vi "LaunchMazeUI.vi"   [LabVIEW 2020]
panel:
  # "Loading Maze UI..."
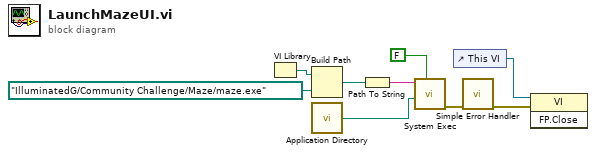
[diagram p0: block diagram]
diagram:
  n1 = VI Library() -> (path=w9:path)
  n2 = Build Path(base path=w9, name or relative path=path "IlluminatedG/Community Challenge/Maze/maze.exe") -> (appended path=w5:path)
  n3 = call <vilib>:"Application Directory.vi"() -> ("Application Directory"=w6:path)
  n4 = Path To String(path=w5) -> (string=w4:string)
  n5 = call <vilib>:"System Exec.vi"("wait until completion? (T)"=FALSE, "working directory"=w6, "command line"=w4) -> ("error out"=w3:errorcluster)  [unwired: 5 in, 3 out]
  n6 = control-ref of="This VI"() -> (w1:refnum<vi>)
  n7 = call <vilib>:"Simple Error Handler.vi"("error in (no error)"=w3) -> ("error out"=w2:errorcluster)  [unwired: 4 in, 4 out]
  n8 = invoke class="VI" method="FP.Close"(reference=w1, error in=w2) -> ()  [unwired: 1 in, 3 out]
